vi "PythonNode.vi"() -> ()   [LabVIEW 2018]
panel:
  out "return value":cluster{"Numeric":dbl, "String":string}
  in  "Numeric":dbl=20.0 format="%#_13g"
  in  "String":string="ABC"
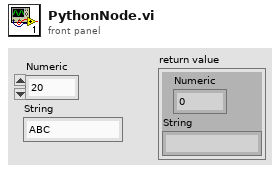
[diagram p1: front panel]
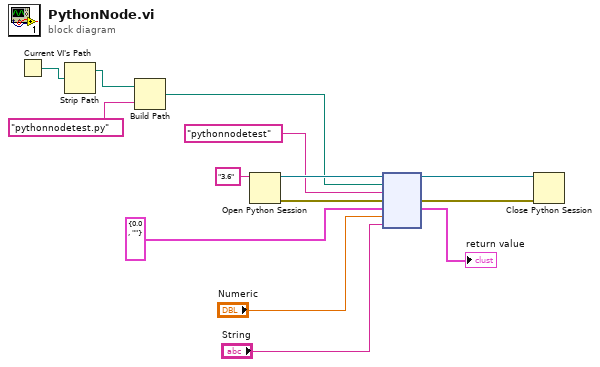
[diagram p0: block diagram]
diagram:
  n1 = Current VI's Path() -> (path=w8:path)
  n2 = Strip Path(path=w8) -> (stripped path=w7:path)  [unwired: 1 out]
  n3 = Build Path(base path=w7, name or relative path="pythonnodetest.py") -> (appended path=w5:path)
  n4 = Open Python Session(python version="3.6" ("Python version")) -> (session out=w14:refnum<k35>, error out=w12:errorcluster)  [unwired: 2 in]
  n5 = node(w14, w5, "pythonnodetest" ("function name"), w12, cluster{"Numeric":dbl, "String":string} {"Numeric"=0.0, "String"=""} ("Cluster"), "Numeric", "String") -> (w13:refnum<k35>, w11:errorcluster, →"return value":cluster{"Numeric":dbl, "String":string})  [unwired: 2 in, 2 out]
  n6 = Close Python Session(session in=w13, error in=w11) -> ()  [unwired: 1 out]
